vi "Servo.vi"() -> ()   [LabVIEW 2014]
uses:
  <vilib>/Platform/TimedLoop/XDataNode/timing_clust.ctl
  <vilib>/Platform/TimedLoop/XDataNode/nitl_modes.ctl
  <vilib>/Platform/TimedLoop/XDataNode/wakeup.ctl
  <vilib>/myRIO/Instrument Drivers/Onboard IO/UART/typedef/VISA Configuration.ctl
  <vilib>/Instr/_visa.llb/VISA Configure Serial Port (Instr).vi
  <vilib>/platform/TimedLoop/XDataNode/XDataNode.xnode
  <vilib>/myRIO/Instrument Drivers/Onboard IO/UART/UART.lvlib
  <vilib>/Platform/TimedLoop/XDataNode/XDNodeRunTimeDep.lvlib
panel:
  out "CountRec":u32
  out "CountSend":u32
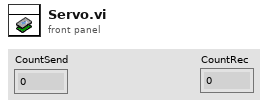
[diagram p1: front panel]
types:
  T1 = typedef "XDNodeRunTimeDep.lvlib/timing_clust.ctl" = cluster{"Expected End [f-1]":u64, "Actual End [f-1]":u64, "Finished Late? [f-1]":bool, "Expected End [i-1]":u64, "Actual End [i-1]":u64, "Finished Late? [i-1]":bool, "Expected Start [i]":u64, "Actual Start [i]":u64, "Expected Start [f]":u64, "Actual Start [f]":u64, "Source Name":string, "Structure Name":string, "Period":i64, "Deadline":i64, "Offset":i64, "Start":i64, "Priority":i32, "Timeout":i32, "Mode":T2, "Wakeup Reason":T3, "Error":errorcluster, "Source Type":string, "Secondary Source Type":string, "Global End Time":u64, "Global Start Time":u64, "Frame Duration":u64, "Iteration Duration":u64, "Assigned CPU":i32, "I/O Scan Engine Mode":u32}
  T2 = typedef "XDNodeRunTimeDep.lvlib/nitl_modes.ctl" = enum32{"No Change", "Process missed periods, maintain original phase", "Discard missed periods, maintain original phase", "Process missed periods, ignore original phase", "Discard missed periods, ignore original phase"}
  T3 = typedef "XDNodeRunTimeDep.lvlib/wakeup.ctl" = enum32{"Normal", "Aborted", "Asynchronous wakeup", "Timing source error", "Timed loop error", "Timeout"}
  T4 = typedef "UART.lvlib/VISA Configuration.ctl" = cluster{"baud rate (9600)":u32, "data bits (8)":u16, "parity (0:none)":enum16{"None", "Odd", "Even", "Mark", "Space"}, "stop bits (10: 1 bit)":u16, "flow control (0:none)":u16, "termination char\n(0xA = '\\n' = LF) ":u8, "Enable Termination\nChar (T)":bool, "timeout (10sec)":u32}
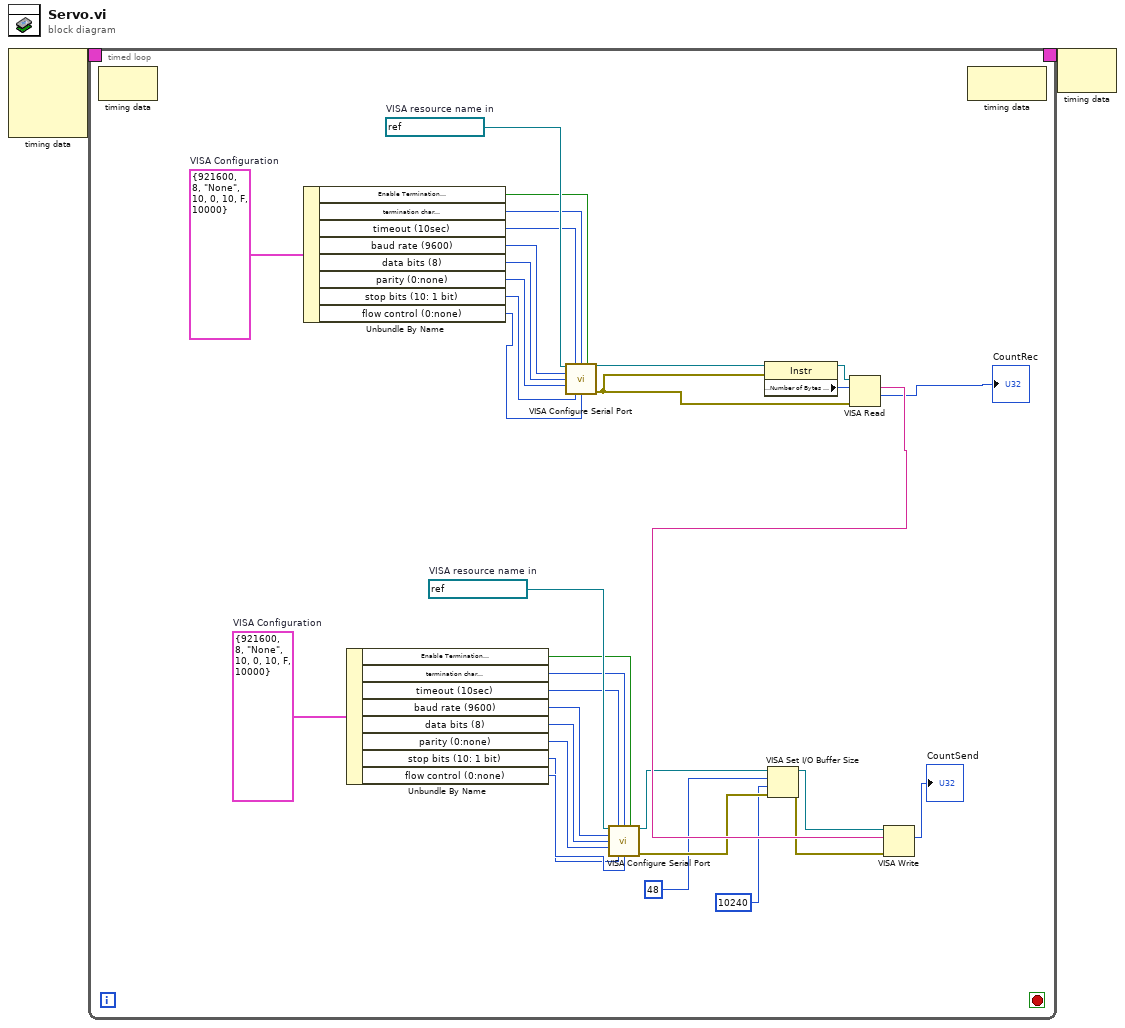
[diagram p0: block diagram]
diagram:
  n1 = node-c288() -> (w2:T1)  [unwired: 4 in]
  n2 = timed-loop {
    timing: w2 -> [_]
    timing-out: [_] -> w1
    stop <- _ stop-if-true
    w22 = T4 {"baud rate (9600)"=921600, "data bits (8)"=8, "parity (0:none)"=enum."None", "stop bits (10: 1 bit)"=10, "flow control (0:none)"=0, "termination char\n(0xA = '\\n' = LF) "=10, "Enable Termination\nChar (T)"=FALSE, "timeout (10sec)"=10000}  # VISA Configuration
    w23 = refnum<visa-resource-name> "ASRL1::INSTR"  # VISA resource name in
    w34 = T4 {"baud rate (9600)"=921600, "data bits (8)"=8, "parity (0:none)"=enum."None", "stop bits (10: 1 bit)"=10, "flow control (0:none)"=0, "termination char\n(0xA = '\\n' = LF) "=10, "Enable Termination\nChar (T)"=FALSE, "timeout (10sec)"=10000}  # VISA Configuration
    w35 = refnum<visa-resource-name> "ASRL1::INSTR"  # VISA resource name in
    n3 = node-c288() -> ()  [unwired: 1 in, 1 out]
    n4 = Unbundle By Name(w34) -> ("Enable Termination\nChar (T)"=w33:bool, "termination char\n(0xA = '\\n' = LF)"=w32:u8, "timeout (10sec)"=w31:u32, "baud rate (9600)"=w26:u32, "data bits (8)"=w27:u16, "parity (0:none)"=w28:enum16{"None", "Odd", "Even", "Mark", "Space"}, "stop bits (10: 1 bit)"=w29:u16, "flow control (0:none)"=w30:u16)
    n5 = Unbundle By Name(w22) -> ("Enable Termination\nChar (T)"=w20:bool, "termination char\n(0xA = '\\n' = LF)"=w19:u8, "timeout (10sec)"=w18:u32, "baud rate (9600)"=w13:u32, "data bits (8)"=w14:u16, "parity (0:none)"=w15:enum16{"None", "Odd", "Even", "Mark", "Space"}, "stop bits (10: 1 bit)"=w16:u16, "flow control (0:none)"=w17:u16)
    n6 = call-poly "VISA Configure Serial Port"("VISA resource name"=w35, "timeout (10sec)"=w31, "termination char\n(0xA = '\\n' = LF)"=w32, "Enable Termination\nChar (T)"=w33, "baud rate (9600)"=w26, "data bits (8)"=w27, "parity (0:none)"=w28, "stop bits (10: 1 bit)"=w29, "flow control (0:none)"=w30) -> ("VISA resource name out"=w4:refnum<visa-resource-name>, "error out"=w3:errorcluster)  [unwired: 5 in]
    n7 = call-poly "VISA Configure Serial Port"("VISA resource name"=w23, "timeout (10sec)"=w18, "termination char\n(0xA = '\\n' = LF)"=w19, "Enable Termination\nChar (T)"=w20, "baud rate (9600)"=w13, "data bits (8)"=w14, "parity (0:none)"=w15, "stop bits (10: 1 bit)"=w16, "flow control (0:none)"=w17) -> ("VISA resource name out"=w9:refnum<visa-resource-name>, "error out"=w8:errorcluster)  [unwired: 5 in]
    n8 = property class="Instr"(reference=w4, error in=w3) -> (reference out=w24:refnum<visa-resource-name>, "Serial Settings:Number of Bytes at Serial Port"=w25:u32)  [unwired: 1 out]
    n9 = VISA Set I/O Buffer Size(VISA resource name=w9, mask (16)=48, size (4096)=10240, error in (no error)=w8) -> (VISA resource name out=w10:refnum<visa-resource-name>, error out=w7:errorcluster)
    n10 = VISA Read(VISA resource name=w24, byte count=w25, error in (no error)=w3) -> (read buffer=w12:string, return count=→"CountRec":u32)  [unwired: 2 out]
    n11 = VISA Write(VISA resource name=w10, write buffer=w12, error in (no error)=w7) -> (return count=→"CountSend":u32)  [unwired: 2 out]
    n12 = node-c288() -> ()  [unwired: 1 in, 1 out]
  }
  n13 = node-c288(w1) -> ()  [unwired: 1 out]
